vi "cblas zgeru.vi"(0 "x":cdb[](array[numeric]), 1 "y":cdb[](array[numeric]), 2 "A":T1, 3 "alpha":cdb=1.0+0.0i, 5 "order":T2=101 items=["CblasRowMajor"=101, "CblasColMajor"=102], 8 "lda":i32, 9 "m":i32=-1, 10 "incx":i32=1, 11 "n":i32=-1, 12 "incy":i32=1) -> (14 "zgeru":T1, 19 "error":i32)   [LabVIEW 2024, in "NI_AALBLAS.lvlib"]
uses:
  NI_AALBLAS.lvlib
  ComplexMatrix.ctl
  Order.ctl
  Operation_Conjugate.ctl
  NI_Matrix.lvlib
  <resource>/lvblas.dll
panel:
  # "void cblas_zgeru(order, m, n, *alpha, *x, incx, *y, incy, *A, lda)"
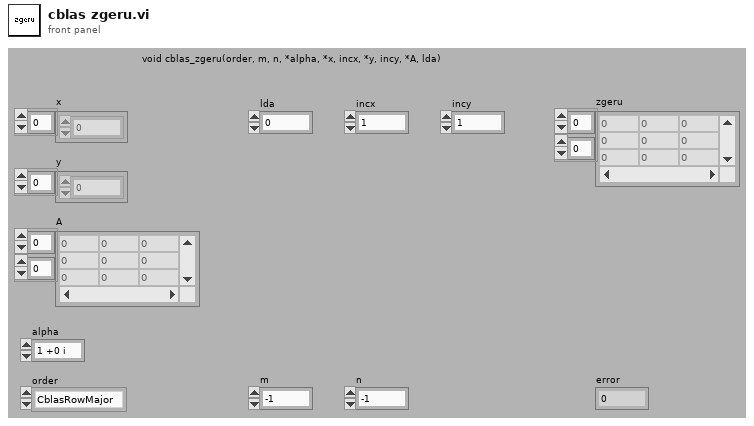
[diagram p1: front panel]
types:
  T1 = typedef "NI_Matrix.lvlib/ComplexMatrix.ctl" = cdb[][]
  T2 = typedef "NI_AALBLAS.lvlib/Order.ctl" = i32
  T3 = typedef "NI_AALBLAS.lvlib/Operation_Conjugate.ctl" = i32
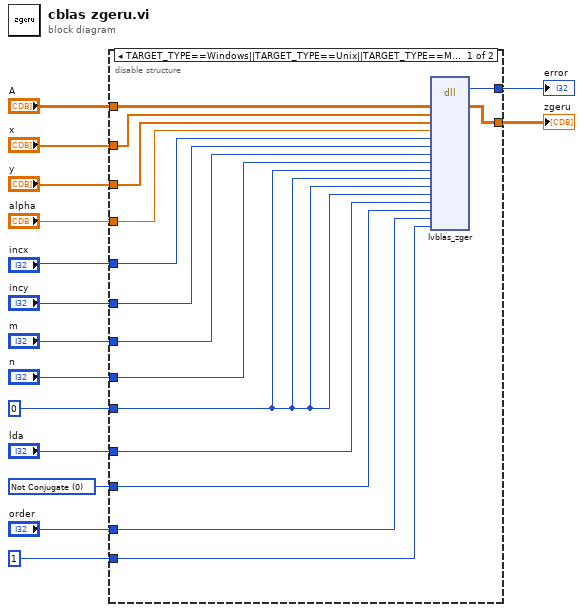
[diagram p0: block diagram]
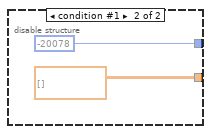
[diagram p2: hidden frame]
diagram:
  w8 = T3 0 items=["Not Conjugate", "Conjugate"] ("operation X")
  n1 = disable-structure shown="TARGET_TYPE==Windows||TARGET_TYPE==Unix||TARGET_TYPE==Mac||TARGET_TYPE==RT" {
    disable-tunnel: "x" -> [w30 _]
    disable-tunnel: "y" -> [w29 _]
    disable-tunnel: "alpha" -> [w21 _]
    disable-tunnel: [w23 T1 [] ("a")] -> w1
    disable-tunnel: "A" -> [w28 _]
    disable-tunnel: [w27 -20078 ("error")] -> w11
    disable-tunnel: 0 -> [w26 _]
    disable-tunnel: "lda" -> [w25 _]
    disable-tunnel: w8 -> [w24 _]
    disable-tunnel: "order" -> [w22 _]
    disable-tunnel: "incx" -> [w20 _]
    disable-tunnel: "incy" -> [w19 _]
    disable-tunnel: "m" -> [w18 _]
    disable-tunnel: "n" -> [w17 _]
    disable-tunnel: 1 -> [w16 _]
    frame condition #0 (active) {
      n2 = dll-call lib="C:/Program Files (x86)/National Instruments/LabVIEW 2024/resource/lvblas.*" fn="lvblas_zger" ("CBLAS.dll:MtrxxVectH")("a"=w28, "x"=w30, "y"=w29, "alpha"=w21, "IncX"=w20, "IncY"=w19, "m"=w18, "n"=w17, "startARow"=w26, "startACol"=w26, "startX"=w26, "startY"=w26, "lda"=w25, "method"=w24, "order"=w22, "check"=w16) -> ("error"=w27:i32, "a"=w23:T1)  [unwired: 18 in, 2 out]
    }
    frame condition #1 {
    }
  }
  "error" <- w11
  "zgeru" <- w1
